vi "Insert Coded Error.vi"(4 "error in (no error)":errorcluster, 5 "non-standard source (\"\")":string, 6 "Reserved Error Code":i32) -> (0 "error out":errorcluster)   [LabVIEW 2013]
doc: "Wire \"Reserved error code\" with an error code output of a LabVIEW function such as the signal generation functions. Error inserted if code is non-zero only.\n\nFreeware from Moore Good Ideas, www.mooregoodideas.com. Do not remove this line."
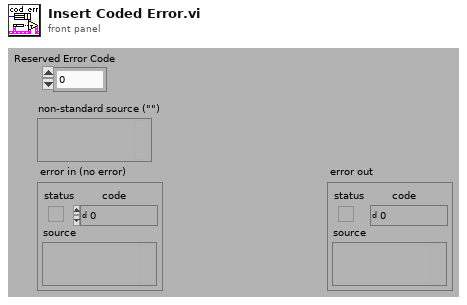
[diagram p1: front panel]
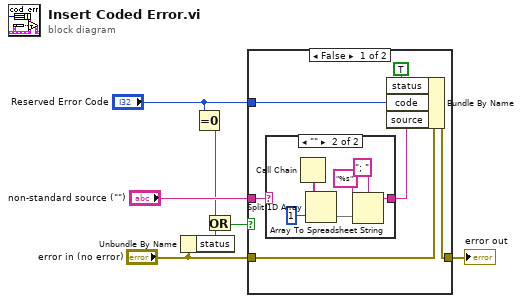
[diagram p0: block diagram]
diagram:
  n1 = Unbundle By Name("error in (no error)") -> ("status"=w4:bool)
  n2 = Equal To 0?(x="Reserved Error Code") -> (x = 0?=w2:bool)
  n3 = Or(x=w2, y=w4) -> (x .or. y?=w3:bool)
  n4 = case shown="False" w3 {
    tunnel: "error in (no error)" -> [w12 w21]
    tunnel: [w9 w21] -> w6
    tunnel: "non-standard source (\"\")" -> [w13 _]
    tunnel: "Reserved Error Code" -> [w8 _]
    frame False {
      n5 = case shown="\"\"" w13 {
        selector: w13 -> [w14 _]
        tunnel: [w14 w15] -> w11
        frame Default {
        }
        frame "" {
          n6 = Call Chain() -> (call chain=w19:string[])
          n7 = Split 1D Array(array=w19, index=1) -> (second subarray=w17:string[])  [unwired: 1 out]
          n8 = Array To Spreadsheet String(delimiter (Tab)="; ", array=w17, 3:"%s" ("format string")) -> (spreadsheet string=w15:string)
        }
      }
      n9 = Bundle By Name(cluster=w12, "status"=TRUE ("Bundle Element"), "code"=w8, "source"=w11) -> (w9:errorcluster)
    }
    frame True {
    }
  }
  "error out" <- w6
